vi "For Loop Progress Bar.vi"(4 "Wait Time (ms)":u32=1000, 6 "Message":string, 7 "Total Iter":i32, 8 "error in (no error)":errorcluster, 10 "Current Iter":i32) -> (0 "error out":errorcluster)   [LabVIEW 2016]
panel:
  out "Progress Bar":dbl(slide) scale=0.0..1.0
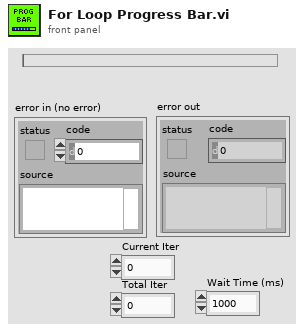
[diagram p1: front panel]
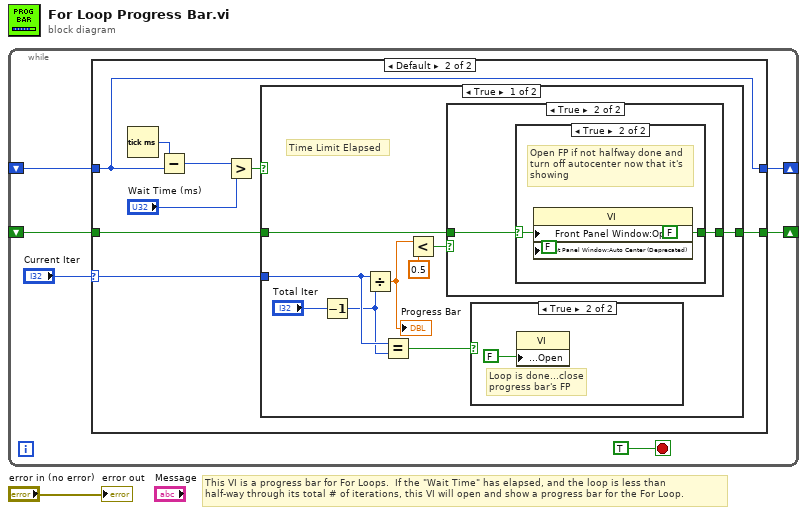
[diagram p0: block diagram]
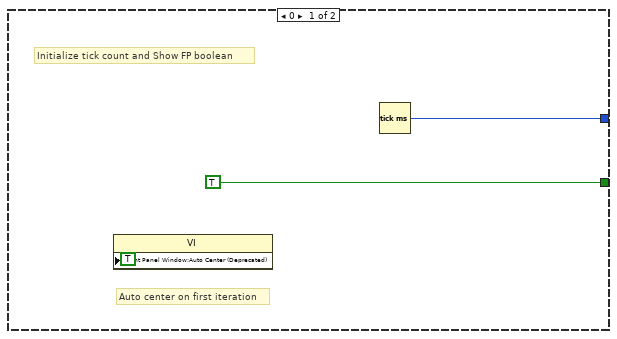
[diagram p2: hidden frame]
diagram:
  # "This VI is a progress bar for For Loops.  If the \"Wait Time\" has elapsed, and the loop is less than\nhalf-way through its total # of iterations, this VI will open and show a progress bar for the For Loop."
  n1 = while {
    shift-right: [w4] -> _
    shift-left: _ -> [w5]
    shift-right: [w2] -> _
    shift-left: _ -> [w3]
    stop <- TRUE stop-if-true
    n2 = case shown="Default" "Current Iter" {
      selector: "Current Iter" -> [_ w16]
      tunnel: w5 -> [_ w17]
      tunnel: [w10 w17] -> w4
      tunnel: w3 -> [_ w15]
      tunnel: [TRUE w14] -> w2
      frame 0 {
        # "Auto center on first iteration"
        # "Initialize tick count and Show FP boolean"
        n3 = property class="VI"("Front Panel Window:Auto Center (Deprecated)"=TRUE ("Front Panel Window:Auto Center")) -> ()  [unwired: 2 in, 2 out]
        n4 = Tick Count (ms)() -> (millisecond timer value=w10:u32)
      }
      frame Default {
        n5 = Tick Count (ms)() -> (millisecond timer value=w18:u32)
        n6 = Subtract(x=w18, y=w17) -> (x-y=w13:u32)
        n7 = Greater?(x=w13, y="Wait Time (ms)") -> (0:w12:bool)
        n8 = case shown="True" w12 {
          tunnel: w16 -> [w23 _]
          tunnel: w15 -> [w25 w36]
          tunnel: [w24 w36] -> w14
          frame True {
            # "Time Limit Elapsed"
            n9 = Decrement(x="Total Iter") -> (x-1=w19:i32)
            n10 = Divide(x=w23, y=w19) -> (x/y=w20:dbl)
            "Progress Bar" <- w20
            n11 = Equal?(x=w23, y=w19) -> (x = y?=w21:bool)
            n12 = Less?(x=w20, y=0.5) -> (x < y?=w27:bool)
            n13 = case shown="True" w27 {
              tunnel: w25 -> [w29 w31]
              tunnel: [w29 w30] -> w24
              frame False {
                # "Progress is over halfway done...just wait it out with no progress bar"
              }
              frame True {
                n14 = case shown="True" w31 {
                  selector: w31 -> [w32 w35]
                  tunnel: [w32 FALSE] -> w30
                  frame False {
                    # "FP has already been opened"
                  }
                  frame True {
                    # "Open FP if not halfway done and turn off autocenter now that it's showing"
                    n15 = property class="VI"("Front Panel Window:Open"=w35, "Front Panel Window:Auto Center (Deprecated)"=FALSE) -> ()  [unwired: 2 in, 2 out]
                  }
                }
              }
            }
            n16 = case shown="True" w21 {
              frame False {
                # "Loop is not done"
              }
              frame True {
                # "Loop is done...close progress bar's FP"
                n17 = property class="VI"("Front Panel Window:Open"=FALSE) -> ()  [unwired: 2 in, 2 out]
              }
            }
          }
          frame False {
            # "Time Limit has not yet elapsed"
          }
        }
      }
    }
  }
  "error out" <- "error in (no error)"
